vi "Read (Multiple Points).vi"(8 "error in (no error)":errorcluster, 9 "Timeout (10000 ms)":i32=10000 format="%#.6g", 11 "VISA resource name":refnum<visa-resource-name>) -> (0 "error out":errorcluster, 2 "Measurements":dbl[](array[numeric])=[2e-06, 2e-06, 2e-06, 2e-06], 3 "VISA resource name out":refnum<visa-resource-name>)   [LabVIEW 2021, in "GWInstek  GDM8351.lvlib"]
doc: "Reads and returns multiple measurements from the instrument. Use this VI when you want to take multiple measurements using an immediate trigger. Use the low-level VIs for other triggering options."
uses:
  <instrlib>/GWInstek  GDM8351/GWInstek  GDM8351.lvlib
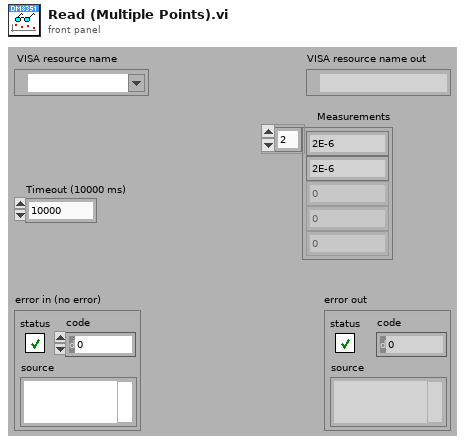
[diagram p1: front panel]
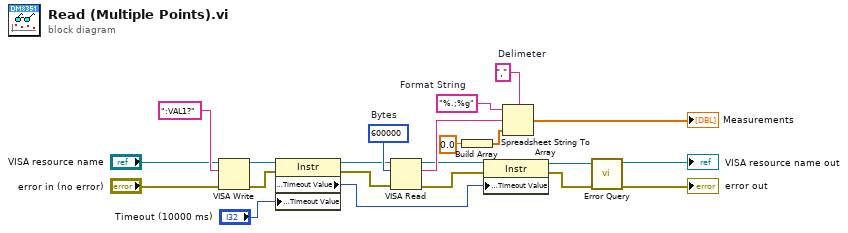
[diagram p0: block diagram]
diagram:
  w17 = ","  # Delimeter
  w18 = "%.;%g"  # Format String
  w22 = u32 600000  # Bytes
  n1 = VISA Write(VISA resource name="VISA resource name", write buffer=":VAL1?", error in (no error)="error in (no error)") -> (VISA resource name out=w13:refnum<visa-resource-name>, error out=w12:errorcluster)  [unwired: 1 out]
  n2 = property class="Instr"(reference=w13, error in=w12, "General Settings:Timeout Value"="Timeout (10000 ms)") -> (reference out=w11:refnum<visa-resource-name>, error out=w10:errorcluster, "General Settings:Timeout Value"=w4:u32)
  n3 = VISA Read(VISA resource name=w11, byte count=w22, error in (no error)=w10) -> (VISA resource name out=w8:refnum<visa-resource-name>, read buffer=w19:string, error out=w6:errorcluster)  [unwired: 1 out]
  n4 = Build Array(0.0) -> (w15:dbl[])
  n5 = property class="Instr"(reference=w8, error in=w6, "General Settings:Timeout Value"=w4) -> (reference out=w7:refnum<visa-resource-name>, error out=w5:errorcluster)
  n6 = Spreadsheet String To Array(delimiter (Tab)=w17, format string=w18, spreadsheet string=w19, array type (2D Dbl)=w15) -> (array=→"Measurements":dbl[])
  n7 = call <instrlib>:"Error Query.vi"("error in (no error)"=w5, "VISA resource name"=w7) -> ("error out"=→"error out":errorcluster, "VISA resource name out"=→"VISA resource name out":refnum<visa-resource-name>)  [unwired: 6 in, 2 out]
